vi "FTW-Inbox-Core-Configuration.vi"(5 "Inbox Configuration":string="{\n  \"Address\": \"tcp://127.0.0.1:*\",\n  \"MaxMessageSize\": 100000,\n  \"AdditionalServiceEndpoints\":\n  {\n    \"Primary\": \"tcp://127.0.0.1:*\",\n    \"RemoteClients\": \"ws://*:*\"\n  },\n  \"MessageRoutingRules\":\n  {\n    \"FTW-PoisonPill\":\n    {\n      \"Accept\": true\n    },\n    \"FTW-ActorStatus\":\n    {\n      \"Accept\": true,\n      \"BusyTimeout\": 100,\n      \"ResponseIncludesIdentity\": true,\n      \"ResponseIncludesTimestamp\": true,\n      \"ResponseIncludesRelativeTimer\": true\n    },\n    \"Default\":\n    {\n      \"Accept\": false,\n      \"Reject\": false,\n      \"BusyTimeout\": -1,\n      \"ResponseIncludesIdentity\": true,\n      \"ResponseIncludesTimestamp\": true,\n      \"ResponseIncludesRelativeTimer\": true\n    }\n  }\n}", 11 "error in":errorcluster) -> (4 "Message Routing Rules":T1[](array[typedef]) {"SendTimeout" format="%dmsec"; "BusyTimeout" format="%dmsec"}, 6 "Additional Endpoint Addresses":string[](array[string]), 8 "Receive Message Size Limit":i32=1000 format="%_4pbytes", 10 "AdditionalServiceEndpoints":string, 15 "error out":errorcluster)   [LabVIEW 2014]
uses:
  FTW-Inbox-Core-RoutingRule.ctl
  lib/FTW-LibraryFilepath.vi
  reflection/FTW-Reflection-Type.vi
  error/FTW-ERR-ThrowGenericError.vi
  error/FTW-ERR-ThrowError.vi
  error/FTW-ERR-NoErrorConstant.vi
  error/FTW-ERR-CallChain.vi
  string/FTW-STR-ReplaceWhitespace.vi
  reflection/FTW-Reflection-Array.vi
  json/core/FTW-JSON-Core-GetFlattenedValue.vi
  json/FTW-JSON-Deserialize/FTW-JSON-Deserialize.xnode
panel:
  # "Inputs"
  # "Outputs"
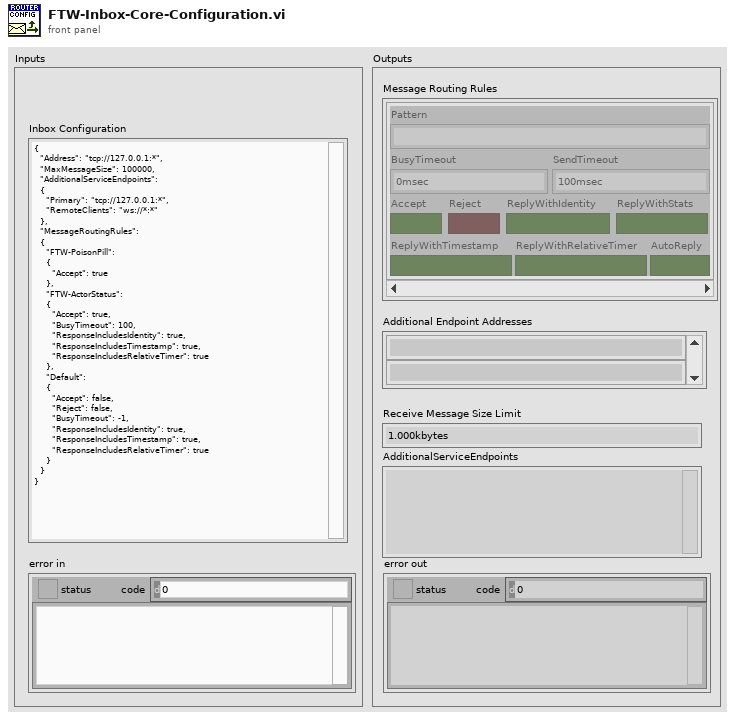
[diagram p1: front panel]
types:
  T1 = typedef "FTW-Inbox-Core-RoutingRule.ctl" = cluster{"Pattern":string, "BusyTimeout":i32, "SendTimeout":i32, "Accept":bool, "Reject":bool, "ReplyWithIdentity":bool, "ReplyWithStats":bool, "ReplyWithTimestamp":bool, "ReplyWithRelativeTimer":bool, "AutoReply":bool}
  T2 = cluster{"MaxMessageSize":i32, "MessageRoutingRules":string, "AdditionalServiceEndpoints":string, "MessageRoutingRules":cluster{"Default":cluster{"Pattern":string, "BusyTimeout":i32, "SendTimeout":i32, "Accept":bool, "Reject":bool, "ReplyWithIdentity":bool, "ReplyWithStatistics":bool, "ReplyWithTimestamp":bool, "ReplyWithRelativeTimer":bool, "AutoReply":bool}, "FTW-PoisonPill":cluster{"Pattern":string, "BusyTimeout":i32, "SendTimeout":i32, "Accept":bool, "Reject":bool, "ReplyWithIdentity":bool, "ReplyWithStatistics":bool, "ReplyWithTimestamp":bool, "ReplyWithRelativeTimer":bool, "AutoReply":bool}, "FTW-ActorStatus":cluster{"Pattern":string, "BusyTimeout":i32, "SendTimeout":i32, "Accept":bool, "Reject":bool, "ReplyWithIdentity":bool, "ReplyWithStatistics":bool, "ReplyWithTimestamp":bool, "ReplyWithRelativeTimer":bool, "AutoReply":bool}}}
  T3 = cluster{"Pattern":string, "BusyTimeout":i32, "SendTimeout":i32, "Accept":bool, "Reject":bool, "ReplyWithIdentity":bool, "ReplyWithStatistics":bool, "ReplyWithTimestamp":bool, "ReplyWithRelativeTimer":bool, "AutoReply":bool}
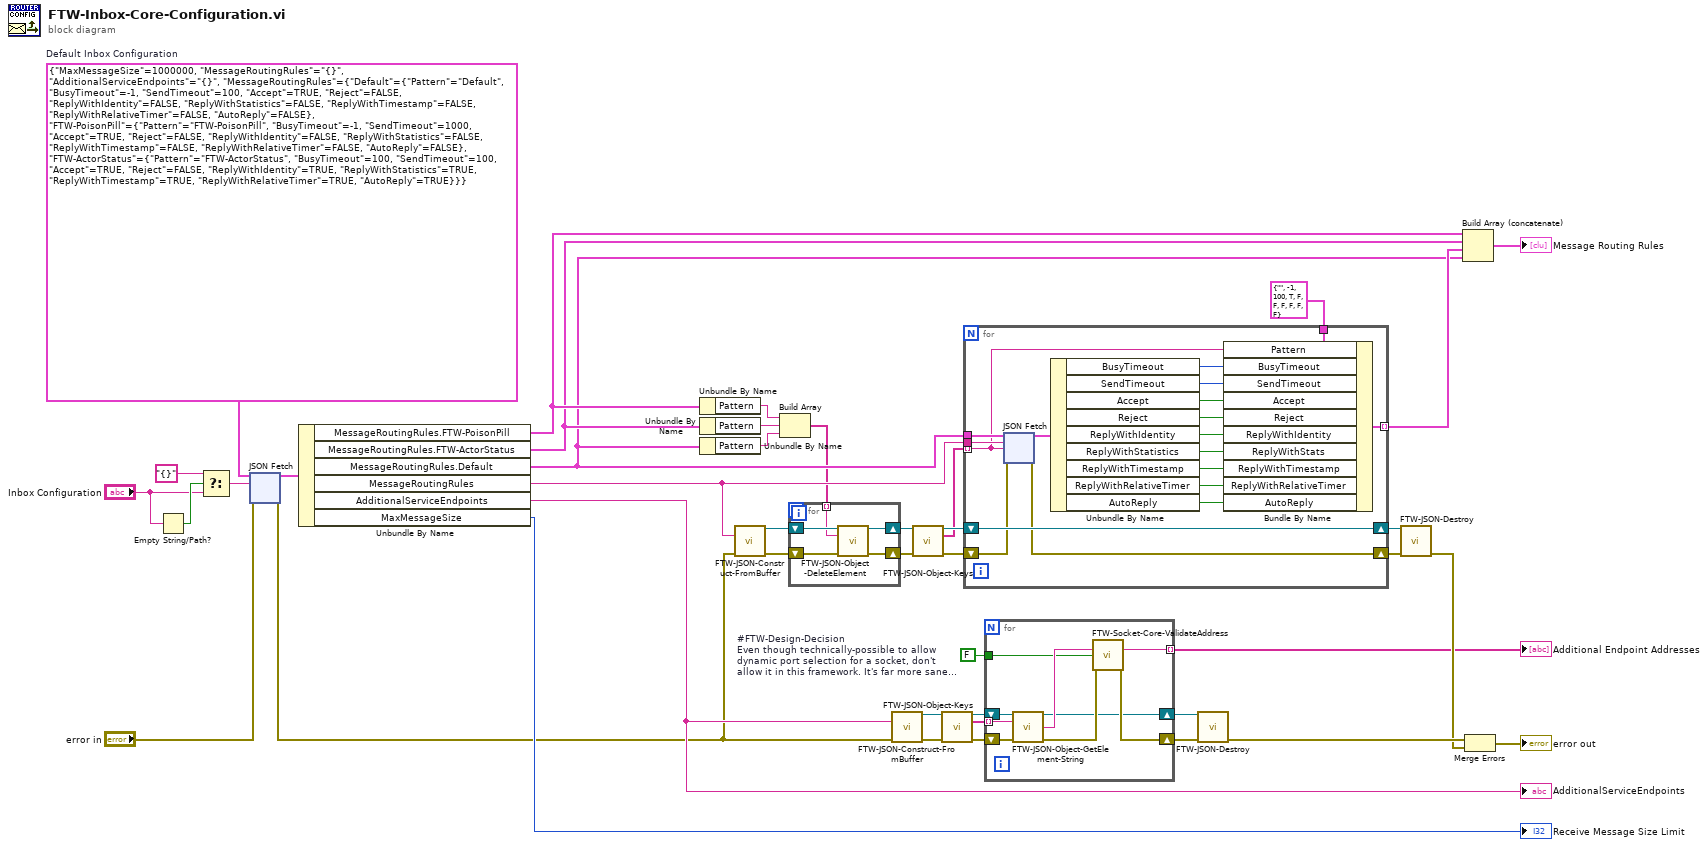
[diagram p0: block diagram]
diagram:
  w14 = FALSE  # #FTW-Design-Decision Even though technically-possible to allow dynamic port selection for a socket, don't allow it in this framework. It's far more sane to fix static addresses agreed upon by all nodes in the system.
  w42 = T2 {"MaxMessageSize"=1000000, "MessageRoutingRules"="{}", "AdditionalServiceEndpoints"="{}", "MessageRoutingRules"={"Default"={"Pattern"="Default", "BusyTimeout"=-1, "SendTimeout"=100, "Accept"=TRUE, "Reject"=FALSE, "ReplyWithIdentity"=FALSE, "ReplyWithStatistics"=FALSE, "ReplyWithTimestamp"=FALSE, "ReplyWithRelativeTimer"=FALSE, "AutoReply"=FALSE}, "FTW-PoisonPill"={"Pattern"="FTW-PoisonPill", "BusyTimeout"=-1, "SendTimeout"=1000, "Accept"=TRUE, "Reject"=FALSE, "ReplyWithIdentity"=FALSE, "ReplyWithStatistics"=FALSE, "ReplyWithTimestamp"=FALSE, "ReplyWithRelativeTimer"=FALSE, "AutoReply"=FALSE}, "FTW-ActorStatus"={"Pattern"="FTW-ActorStatus", "BusyTimeout"=100, "SendTimeout"=100, "Accept"=TRUE, "Reject"=FALSE, "ReplyWithIdentity"=TRUE, "ReplyWithStatistics"=TRUE, "ReplyWithTimestamp"=TRUE, "ReplyWithRelativeTimer"=TRUE, "AutoReply"=TRUE}}}  # Default Inbox Configuration
  n1 = Empty String/Path?(string/path="Inbox Configuration") -> (empty?=w4:bool)
  n2 = Select(t="{}", s=w4, f="Inbox Configuration") -> (s? t:f=w2:string)
  n3 = xnode "JSON Fetch"("Type and Defaults"=w42, "JSON String"=w2, "error in"="error in") -> ("Values"=w40:T2, "error out"=w13:errorcluster)  [unwired: 1 in]
  n4 = Unbundle By Name(w40) -> ("MessageRoutingRules.FTW-PoisonPill"=w11:T3, "MessageRoutingRules.FTW-ActorStatus"=w10:T3, "MessageRoutingRules.Default"=w9:T3, "MessageRoutingRules"=w12:string, "AdditionalServiceEndpoints"=w39:string, "MaxMessageSize"=→"Receive Message Size Limit":i32)
  "AdditionalServiceEndpoints" <- w39
  n5 = Unbundle By Name(w11) -> ("Pattern"=w8:string)
  n6 = Unbundle By Name(w10) -> ("Pattern"=w7:string)
  n7 = Unbundle By Name(w9) -> ("Pattern"=w6:string)
  n8 = call "FTW-JSON-Construct-FromBuffer.vi"("JSON String (UTF-8)"=w12, "error in"=w13) -> ("JSON Object"=w20:refnum<data-value>, "error out"=w18:errorcluster)  [unwired: 12 in]
  n9 = Build Array(w8, w7, w6) -> (w5:string[])
  n10 = for {
    shift-right: [w46] -> w19
    shift-left: w20 -> [w47]
    shift-right: [w44] -> w17
    shift-left: w18 -> [w45]
    tunnel: w5 -> [w43] mode=indexing
    n11 = call "FTW-JSON-Object-DeleteElement.vi"("JSON Object"=w47, "Key"=w43, "error in"=w45) -> ("JSON Object out"=w46:refnum<data-value>, "error out"=w44:errorcluster)  [unwired: 10 in, 1 out]
  }
  n12 = call "FTW-JSON-Construct-FromBuffer.vi"("JSON String (UTF-8)"=w39, "error in"=w13) -> ("JSON Object"=w33:refnum<data-value>, "error out"=w32:errorcluster)  [unwired: 12 in]
  n13 = call "FTW-JSON-Object-Keys.vi"("JSON Object"=w19, "error in"=w17) -> ("JSON Object out"=w28:refnum<data-value>, "Keys"=w27:string[], "error out"=w29:errorcluster)  [unwired: 11 in]
  n14 = call "FTW-JSON-Object-Keys.vi"("JSON Object"=w33, "error in"=w32) -> ("JSON Object out"=w37:refnum<data-value>, "Keys"=w38:string[], "error out"=w36:errorcluster)  [unwired: 11 in]
  n15 = for {
    shift-right: [w61] -> w31
    shift-left: w29 -> [w62]
    tunnel: w27 -> [w51] mode=indexing
    shift-right: [w63] -> w30
    shift-left: w28 -> [w63]
    tunnel: w9 -> [w65]
    tunnel: w12 -> [w64]
    tunnel: [w58] -> w15 mode=indexing
    tunnel: T1 {"Pattern"="", "BusyTimeout"=-1, "SendTimeout"=100, "Accept"=TRUE, "Reject"=FALSE, "ReplyWithIdentity"=FALSE, "ReplyWithStats"=FALSE, "ReplyWithTimestamp"=FALSE, "ReplyWithRelativeTimer"=FALSE, "AutoReply"=FALSE} ("Routing Rule") -> [w59]
    n16 = xnode "JSON Fetch"("Type and Defaults"=w65, "JSON String"=w64, "Element Path"=w51, "error in"=w62) -> ("Values"=w60:T3, "error out"=w61:errorcluster)
    n17 = Unbundle By Name(w60) -> ("BusyTimeout"=w57:i32, "SendTimeout"=w56:i32, "Accept"=w55:bool, "Reject"=w54:bool, "ReplyWithIdentity"=w53:bool, "ReplyWithStatistics"=w52:bool, "ReplyWithTimestamp"=w50:bool, "ReplyWithRelativeTimer"=w49:bool, "AutoReply"=w48:bool)
    n18 = Bundle By Name(cluster=w59, "Pattern"=w51, "BusyTimeout"=w57, "SendTimeout"=w56, "Accept"=w55, "Reject"=w54, "ReplyWithIdentity"=w53, "ReplyWithStats"=w52, "ReplyWithTimestamp"=w50, "ReplyWithRelativeTimer"=w49, "AutoReply"=w48) -> (w58:T1)
  }
  n19 = for {
    tunnel: [w109] -> w21 mode=indexing
    shift-right: [w110] -> w34
    shift-left: w36 -> [w105]
    tunnel: w38 -> [w107] mode=indexing
    shift-right: [w103] -> w35
    shift-left: w37 -> [w108]
    tunnel: w14 -> [w102]
    n20 = call "FTW-JSON-Object-GetElement-String.vi"("JSON Object"=w108, "Key"=w107, "error in"=w105) -> ("JSON Object out"=w103:refnum<data-value>, "Value"=w106:string, "error out"=w104:errorcluster)  [unwired: 9 in, 1 out]
    n21 = call "FTW-Socket-Core-ValidateAddress.vi"("Address"=w106, "Allow wildcard replacement?"=w102, "error in"=w104) -> ("Sanitized Address"=w109:string, "error out"=w110:errorcluster)  [unwired: 10 in, 1 out]
  }
  "Additional Endpoint Addresses" <- w21
  n22 = call "FTW-JSON-Destroy.vi"("JSON Object"=w35, "error in"=w34) -> ("error out"=w26:errorcluster)  [unwired: 13 in]
  n23 = call "FTW-JSON-Destroy.vi"("JSON Object"=w30, "error in"=w31) -> ("error out"=w24:errorcluster)  [unwired: 13 in]
  n24 = Build Array (concatenate)(w11, w10, w15, w9) -> (→"Message Routing Rules":T1[])
  n25 = Merge Errors(w26, w24) -> (→"error out":errorcluster)
